vi "CRYTable Value Change.vi"(4 "Column":i32, 6 "Row":i32, 7 "TableVI":refnum<vi>, 8 "NewVal":string, 9 "OldVal":string, 10 "Index":i32, 11 "Type":enum16{"Curves", "Values", "Results", "WFM"}(ring)) -> ()   [LabVIEW 2013]
uses:
  Control/CRYTable Property.ctl
panel:
  in  "Table Property":T1 {"Precision" items=["Digits of precision", "Significant digits"]}
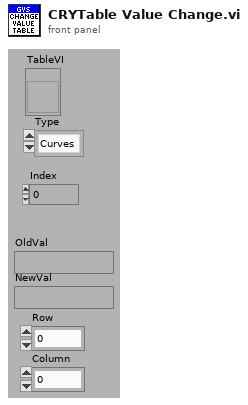
[diagram p1: front panel]
types:
  T1 = typedef "CRYTable Property.ctl" = cluster{"Reset All Columns":bool, "Transpose":bool, "Display Units":bool, "Notation":u16, "Digits":u16, "Precision":u16, "Hide Traling Zeros":bool, "Column Width":u16, "Row Header Width":u16, "Show vertical scroll bar":bool, "Show horizontal scroll bar":bool}
  T2 = enum16{"OK", "Yes", "YesNo", "YesNoCancel", "ReplaceAppend"}
  T3 = typedef "CRYData Cluster.ctl" = cluster{"Name":string, "Curve":cluster{"x":dbl, "y":dbl, "z":dbl}[], "X data":u16, "Y data":u16, "Z data":u16, "X axis":u16, "Y axis":u16, "Z axis":u16, "X unit":string, "Y unit":string, "Z unit":string, "X dB ref":dbl, "Y dB ref":dbl, "Z dB ref":dbl, "single val":bool, "protected":bool, "display X":bool, "display Y":bool, "display Z":bool, "Test Info":string, "Step No.":i32, "Plot Settings":cluster{"Color":u32, "Interpolation":u8, "Point Style":u8, "Line Style":u8, "Point Color":u32, "Line Width":u8, "Bar Plot Style":u8, "Fill To":i16}, "AutoProtect":bool}
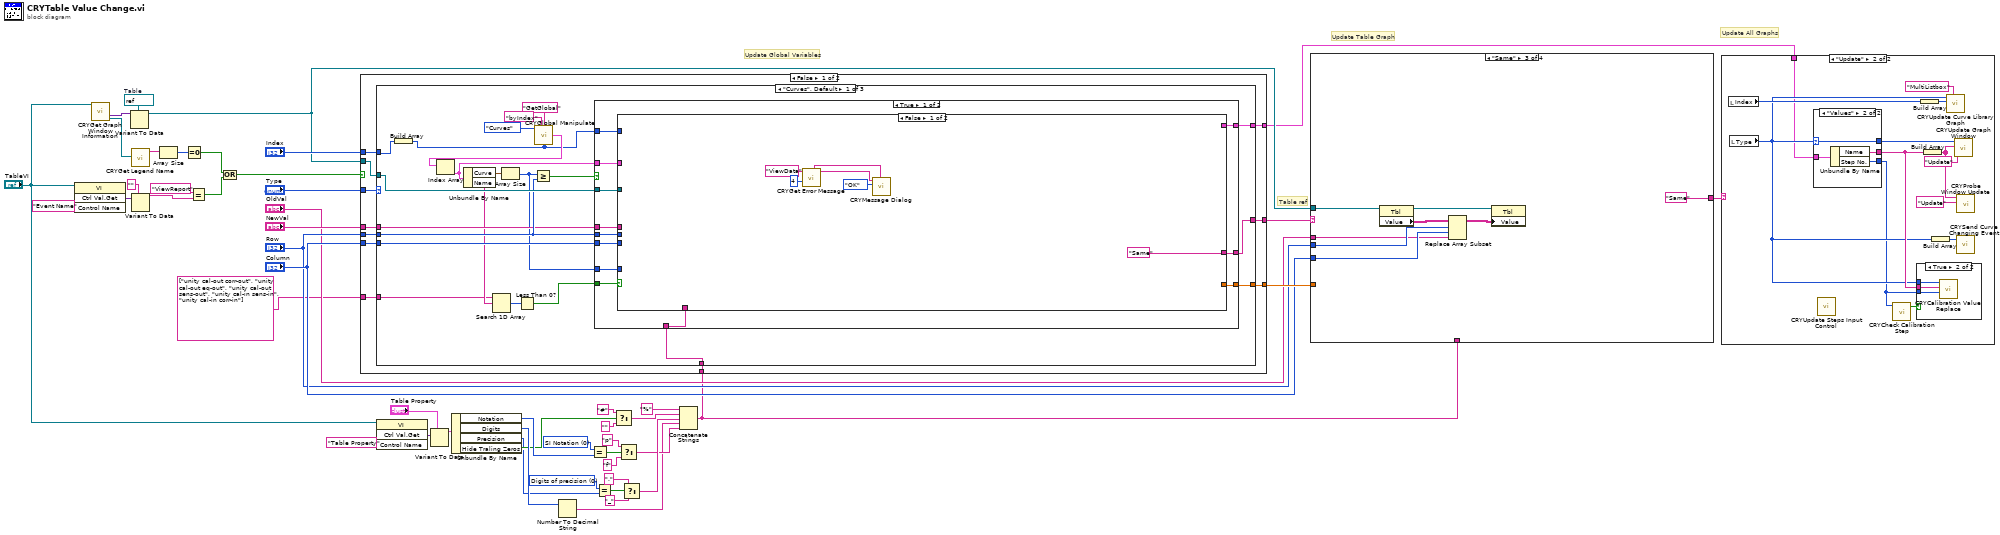
[diagram p0: block diagram]
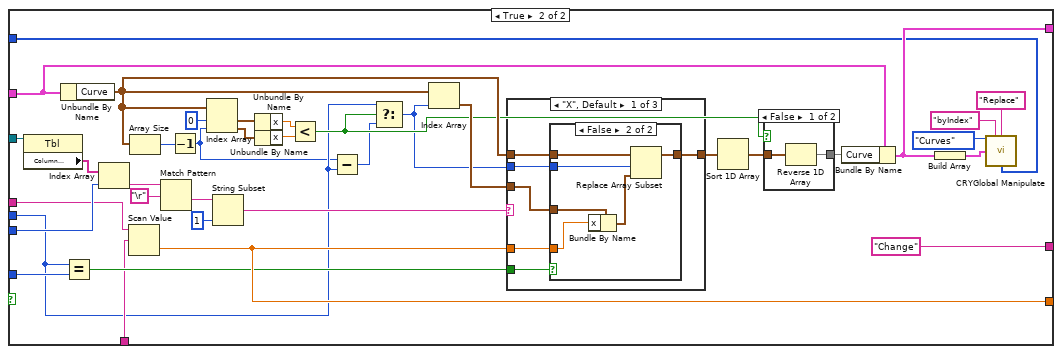
[diagram p2: hidden frame]
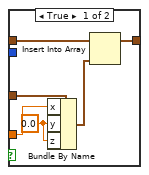
[diagram p4: hidden frame]
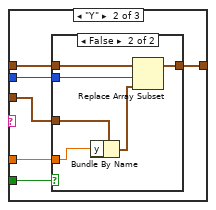
[diagram p5: hidden frame]
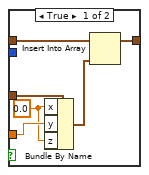
[diagram p6: hidden frame]
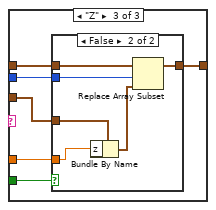
[diagram p7: hidden frame]
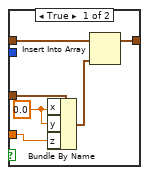
[diagram p8: hidden frame]
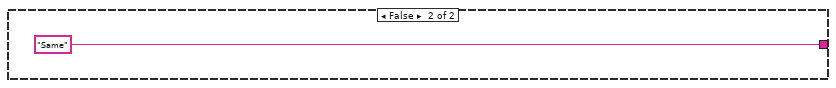
[diagram p9: hidden frame]
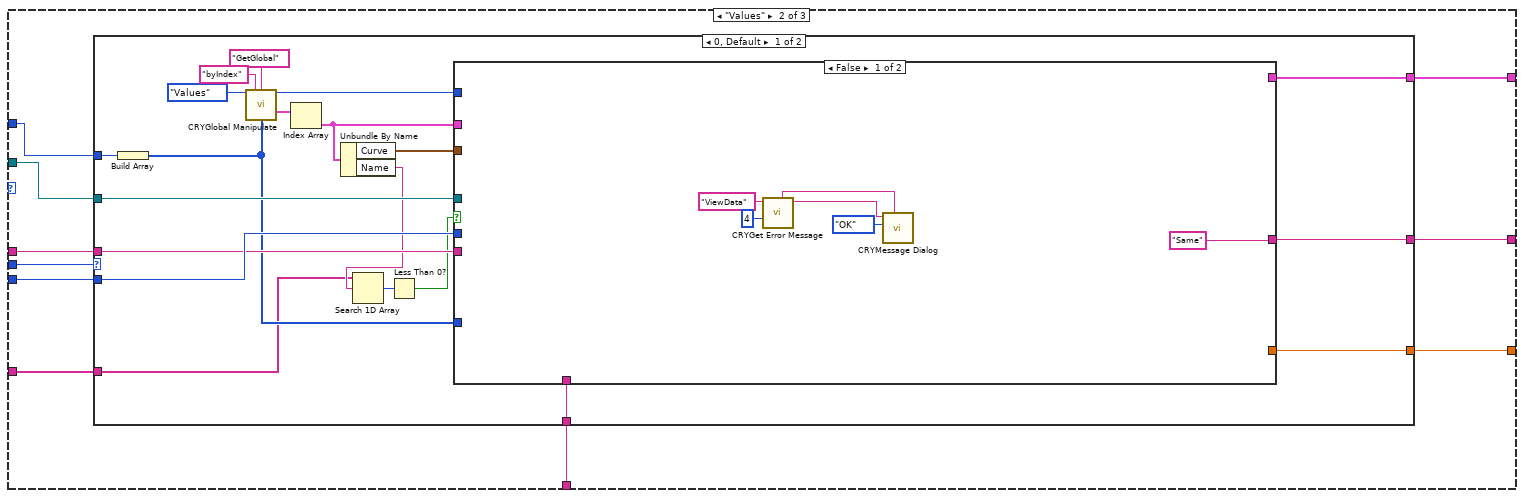
[diagram p10: hidden frame]
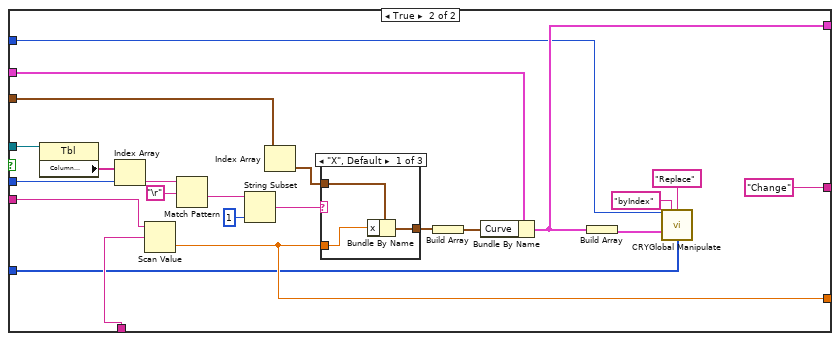
[diagram p11: hidden frame]
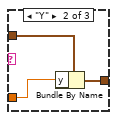
[diagram p12: hidden frame]
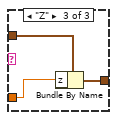
[diagram p13: hidden frame]
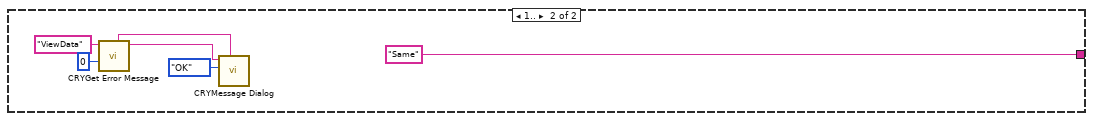
[diagram p14: hidden frame]
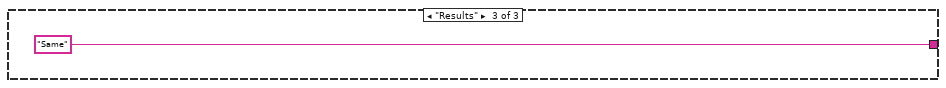
[diagram p15: hidden frame]
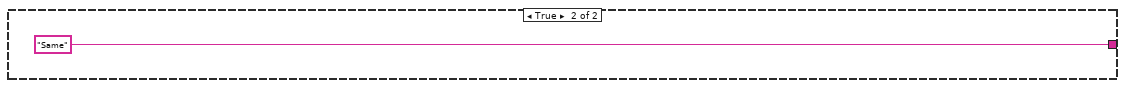
[diagram p16: hidden frame]
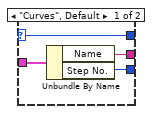
[diagram p19: hidden frame]
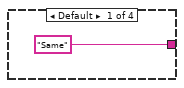
[diagram p20: hidden frame]
diagram:
  w31 = u16 0 items=["Digits of precision", "Significant digits"] ("Precision")
  w32 = u16 0 items=["SI Notation", "Floating point"] ("Notation")
  w48 = refnum<vi> refnum  # Table
  # "Table ref"
  # "Update All Graphs"
  # "Update Table Graph"
  # "Update Global Variables"
  n1 = invoke class="VI" method="Ctrl Val.Get"(reference="TableVI", "Control Name"="Event Name") -> ("Get Control Value Variant"=w14:variant)  [unwired: 2 in, 3 out]
  n2 = call "CRYGet Graph Window Information.vi"("pGraph VI In"="TableVI") -> ("Graph Control Ref Out"=w47:variant, "Legend Ref Out"=w11:refnum<vi>)  [unwired: 4 in, 9 out]
  n3 = Variant To Data(type=w48, Variant=w47) -> (data=w3:refnum<vi>)  [unwired: 1 in, 1 out]
  n4 = call "CRYGet Legend Name.vi"("MCListbox Refnum"=w11) -> ("Names Out"=w8:string[])  [unwired: 10 in]
  n5 = Variant To Data(type="" ("Control Name"), Variant=w14) -> (data=w10:string)  [unwired: 1 in, 1 out]
  n6 = Array Size(array=w8) -> (size(s)=w7:i32)
  n7 = Equal To 0?(x=w7) -> (x = 0?=w6:bool)
  n8 = Equal?(x="ViewReport", y=w10) -> (x = y?=w5:bool)
  n9 = Or(x=w6, y=w5) -> (x .or. y?=w4:bool)
  n10 = invoke class="VI" method="Ctrl Val.Get"(reference="TableVI", "Control Name"="Table Property") -> ("Get Control Value Variant"=w39:variant)  [unwired: 2 in, 3 out]
  n11 = Variant To Data(type="Table Property", Variant=w39) -> (data=w37:T1)  [unwired: 1 in, 1 out]
  n12 = Unbundle By Name(w37) -> ("Notation"=w35:u16, "Digits"=w36:u16, "Precision"=w33:u16, "Hide Traling Zeros"=w34:bool)
  n13 = Number To Decimal String(number=w36) -> (decimal integer string=w18:string)  [unwired: 1 in]
  n14 = Equal?(x=w32, y=w35) -> (x = y?=w29:bool)
  n15 = Equal?(x=w31, y=w33) -> (x = y?=w23:bool)
  n16 = Select(t="#" ("format string"), s=w34, f="" ("format string")) -> (s? t:f=w24:string)
  n17 = Select(t="p" ("string"), s=w29, f="f" ("string")) -> (s? t:f=w19:string)
  n18 = Select(t=".", s=w23, f="_") -> (s? t:f=w22:string)
  n19 = Concatenate Strings("%" ("string"), w24, w22, w18, w19) -> (w16:string)
  n20 = case shown="False" w4 {
    tunnel: [w61 _] -> w50
    tunnel: [w60 "Same" ("output string")] -> w49
    tunnel: w3 -> [w59 _]
    tunnel: "Column" -> [w58 _]
    tunnel: "Row" -> [w57 _]
    tunnel: "Type" -> [w56 _]
    tunnel: "Index" -> [w55 _]
    tunnel: "NewVal" -> [w54 _]
    tunnel: w16 -> [w53 _]
    tunnel: [w52 _] -> w2
    tunnel: string[] ["unity cal-out corr-out", "unity cal-out eq-out", "unity cal-out sens-out", "unity cal-in sens-in", "unity cal-in corr-in"] ("item tags") -> [w51 _]
    frame False {
      n21 = case shown="\"Curves\", Default" w56 {
        tunnel: w57 -> [w80 w204 _]
        tunnel: w58 -> [w83 w206 _]
        tunnel: w59 -> [w82 w205 _]
        tunnel: w55 -> [w74 w203 _]
        tunnel: [w79 w202 _] -> w61
        tunnel: [w78 w201 "Same" ("output string")] -> w60
        tunnel: w54 -> [w77 w200 _]
        tunnel: w53 -> [w75 w199 _]
        tunnel: [w71 w198 _] -> w52
        tunnel: w51 -> [w65 w197 _]
        frame "Curves", Default {
          n22 = Build Array(w74) -> (w67:i32[])
          n23 = call "CRYGlobal Manipulate.vi"("Type"=enum16{"Curves", "Values", "Results", "WFM"}."Curves", "sOption"="byIndex", "sAction"="GetGlobal", "nData"=w67) -> ("Curves Out"=w73:T3[])  [unwired: 5 in, 6 out]
          n24 = Index Array(array=w73) -> (element=w72:T3)  [unwired: 1 in]
          n25 = Unbundle By Name(w72) -> ("Curve"=w81:cluster{"x":dbl, "y":dbl, "z":dbl}[], "Name"=w66:string)
          n26 = Search 1D Array(1D array=w65, element=w66) -> (index of element=w64:i32)  [unwired: 1 in]
          n27 = Array Size(array=w81) -> (size(s)=w76:i32)
          n28 = Less Than 0?(x=w64) -> (x < 0?=w62:bool)
          n29 = Greater Or Equal?(x=w76, y=w80) -> (x >= y?=w63:bool)
          n30 = case shown="True" w63 {
            tunnel: w80 -> [w88 _]
            tunnel: w83 -> [w95 _]
            tunnel: w82 -> [w94 _]
            tunnel: [w93 _] -> w79
            tunnel: [w90 "Same" ("output string")] -> w78
            tunnel: w77 -> [w92 _]
            tunnel: w76 -> [w91 _]
            tunnel: w75 -> [w89 _]
            tunnel: w72 -> [w87 _]
            tunnel: w67 -> [w85 _]
            tunnel: [w86 _] -> w71
            tunnel: w62 -> [w84 _]
            frame True {
              n31 = case shown="False" w84 {
                tunnel: w95 -> [_ w137]
                tunnel: w94 -> [_ w133]
                tunnel: [_ w129] -> w93
                tunnel: w92 -> [_ w128]
                tunnel: w91 -> [_ w127]
                tunnel: ["Same" ("output string") "Change" ("output string")] -> w90
                tunnel: w89 -> [_ w124]
                tunnel: w88 -> [_ w113]
                tunnel: w87 -> [_ w105]
                tunnel: [_ w104] -> w86
                tunnel: w85 -> [_ w103]
                frame False {
                  n32 = call "CRYGet Error Message.vi"("Error No"=4, "Kind"="ViewData") -> ("Message"=w96:string, "Window Title"=w97:string)  [unwired: 4 in, 4 out]
                  n33 = call "CRYMessage Dialog.vi"("Window Title"=w97, "YesNoCancel"=T2."OK", "Message Content"=w96) -> ()  [unwired: 7 in, 2 out]
                }
                frame True {
                  n34 = property on="Property Node" class="Tbl"(reference=w133) -> ("Column Headers[]"=w138:string[])  [unwired: 1 in, 2 out]
                  n35 = Unbundle By Name(w105) -> ("Curve"=w123:cluster{"x":dbl, "y":dbl, "z":dbl}[])
                  n36 = Equal?(x=w113, y=w127) -> (x = y?=w126:bool)
                  n37 = Index Array(array=w138, index=w137) -> (element=w131:string)
                  n38 = Scan Value(string=w128, format string=w124) -> (value=w129:dbl)  [unwired: 1 in, 1 out]
                  n39 = Array Size(array=w123) -> (size(s)=w111:i32)
                  n40 = Match Pattern(string=w131, regular expression="\r") -> (after substring=w130:string)  [unwired: 1 in, 3 out]
                  n41 = Decrement(x=w111) -> (x-1=w109:i32)
                  n42 = Index Array(array=w123, index #1=0 ("index"), index #2=w109) -> (element #1=w121:cluster{"x":dbl, "y":dbl, "z":dbl}, element #2=w120:cluster{"x":dbl, "y":dbl, "z":dbl})
                  n43 = String Subset(string=w130, length (rest)=1 ("length (rest)")) -> (substring=w135:string)  [unwired: 1 in]
                  n44 = Unbundle By Name(w121) -> ("x"=w119:dbl)
                  n45 = Unbundle By Name(w120) -> ("x"=w118:dbl)
                  n46 = Less?(x=w119, y=w118) -> (x < y?=w114:bool)
                  n47 = Subtract(x=w109, y=w113) -> (x-y=w112:i32)
                  n48 = Select(t=w113, s=w114, f=w112) -> (s? t:f=w110:i32)
                  n49 = Index Array(array=w123, index=w110) -> (element=w134:cluster{"x":dbl, "y":dbl, "z":dbl})
                  n50 = case shown="\"X\", Default" w135 {
                    tunnel: w134 -> [w145 w163 w181]
                    tunnel: w129 -> [w147 w165 w183]
                    tunnel: w123 -> [w144 w162 w180]
                    tunnel: w110 -> [w143 w161 w179]
                    tunnel: [w142 w160 w178] -> w116
                    tunnel: w126 -> [w146 w164 w182]
                    frame "X", Default {
                      n51 = case shown="False" w146 {
                        tunnel: w147 -> [w153 w159]
                        tunnel: w145 -> [w152 w158]
                        tunnel: w144 -> [w150 w157]
                        tunnel: [w148 w155] -> w142
                        tunnel: w143 -> [_ w154]
                        frame True {
                          w151 = 0.0 ("y")
                          n52 = Bundle By Name(cluster=w152, "x"=w153, "y"=w151, "z"=w151) -> (w149:cluster{"x":dbl, "y":dbl, "z":dbl})
                          n53 = Insert Into Array(array=w150, new element=w149) -> (w148:cluster{"x":dbl, "y":dbl, "z":dbl}[])  [unwired: 1 in]
                        }
                        frame False {
                          n54 = Bundle By Name(cluster=w158, "x"=w159) -> (w156:cluster{"x":dbl, "y":dbl, "z":dbl})
                          n55 = Replace Array Subset(array=w157, new element=w156, index=w154) -> (w155:cluster{"x":dbl, "y":dbl, "z":dbl}[])
                        }
                      }
                    }
                    frame "Y" {
                      n56 = case shown="False" w164 {
                        tunnel: w165 -> [w167 w172]
                        tunnel: w163 -> [w171 w177]
                        tunnel: w162 -> [w170 w176]
                        tunnel: [w168 w174] -> w160
                        tunnel: w161 -> [_ w173]
                        frame True {
                          w166 = 0.0 ("x")
                          n57 = Bundle By Name(cluster=w171, "x"=w166, "y"=w167, "z"=w166) -> (w169:cluster{"x":dbl, "y":dbl, "z":dbl})
                          n58 = Insert Into Array(array=w170, new element=w169) -> (w168:cluster{"x":dbl, "y":dbl, "z":dbl}[])  [unwired: 1 in]
                        }
                        frame False {
                          n59 = Bundle By Name(cluster=w177, "y"=w172) -> (w175:cluster{"x":dbl, "y":dbl, "z":dbl})
                          n60 = Replace Array Subset(array=w176, new element=w175, index=w173) -> (w174:cluster{"x":dbl, "y":dbl, "z":dbl}[])
                        }
                      }
                    }
                    frame "Z" {
                      n61 = case shown="False" w182 {
                        tunnel: w183 -> [w184 w195]
                        tunnel: w181 -> [w189 w194]
                        tunnel: w180 -> [w188 w193]
                        tunnel: [w186 w191] -> w178
                        tunnel: w179 -> [_ w190]
                        frame True {
                          w185 = 0.0 ("y")
                          n62 = Bundle By Name(cluster=w189, "x"=w185, "y"=w185, "z"=w184) -> (w187:cluster{"x":dbl, "y":dbl, "z":dbl})
                          n63 = Insert Into Array(array=w188, new element=w187) -> (w186:cluster{"x":dbl, "y":dbl, "z":dbl}[])  [unwired: 1 in]
                        }
                        frame False {
                          n64 = Bundle By Name(cluster=w194, "z"=w195) -> (w192:cluster{"x":dbl, "y":dbl, "z":dbl})
                          n65 = Replace Array Subset(array=w193, new element=w192, index=w190) -> (w191:cluster{"x":dbl, "y":dbl, "z":dbl}[])
                        }
                      }
                    }
                  }
                  n66 = Sort 1D Array(array=w116) -> (sorted array=w115:cluster{"x":dbl, "y":dbl, "z":dbl}[])
                  n67 = case shown="False" w114 {
                    tunnel: w115 -> [w140 w141]
                    tunnel: [w139 w141] -> w117
                    frame False {
                      n68 = Reverse 1D Array(array=w140) -> (reversed array=w139:cluster{"x":dbl, "y":dbl, "z":dbl}[])
                    }
                    frame True {
                    }
                  }
                  n69 = Bundle By Name(cluster=w105, "Curve"=w117) -> (w104:T3)
                  n70 = Build Array(w104) -> (w106:T3[])
                  n71 = call "CRYGlobal Manipulate.vi"("Type"=enum16{"Curves", "Values", "Results", "WFM"}."Curves", "sOption"="byIndex", "sAction"="Replace", "Curves"=w106, "nData"=w103) -> ()  [unwired: 4 in, 7 out]
                }
              }
            }
            frame False {
            }
          }
        }
        frame "Values" {
          n72 = case shown="0, Default" w204 {
            tunnel: w206 -> [w226 _]
            tunnel: w205 -> [w224 _]
            tunnel: w203 -> [w219 _]
            tunnel: [w223 _] -> w202
            tunnel: [w222 "Same" ("output string")] -> w201
            tunnel: w200 -> [w221 _]
            tunnel: w199 -> [w220 _]
            tunnel: [w216 _] -> w198
            tunnel: w197 -> [w208 _]
            frame 0, Default {
              n73 = Build Array(w219) -> (w211:i32[])
              n74 = call "CRYGlobal Manipulate.vi"("Type"=enum16{"Curves", "Values", "Results", "WFM"}."Values", "sOption"="byIndex", "sAction"="GetGlobal", "nData"=w211) -> ("Type out"=w213:enum16{"Curves", "Values", "Results", "WFM"}, "Values Out"=w218:T3[])  [unwired: 5 in, 5 out]
              n75 = Index Array(array=w218) -> (element=w217:T3)  [unwired: 1 in]
              n76 = Unbundle By Name(w217) -> ("Curve"=w225:cluster{"x":dbl, "y":dbl, "z":dbl}[], "Name"=w209:string)
              n77 = Search 1D Array(1D array=w208, element=w209) -> (index of element=w210:i32)  [unwired: 1 in]
              n78 = Less Than 0?(x=w210) -> (x < 0?=w207:bool)
              n79 = case shown="False" w207 {
                tunnel: w226 -> [_ w254]
                tunnel: w225 -> [_ w251]
                tunnel: w224 -> [_ w249]
                tunnel: [_ w243] -> w223
                tunnel: ["Same" ("output string") "Change" ("output string")] -> w222
                tunnel: w221 -> [_ w241]
                tunnel: w220 -> [_ w240]
                tunnel: w217 -> [_ w237]
                tunnel: [_ w236] -> w216
                tunnel: w213 -> [_ w235]
                tunnel: w211 -> [_ w234]
                frame False {
                  n80 = call "CRYGet Error Message.vi"("Error No"=4, "Kind"="ViewData") -> ("Message"=w227:string, "Window Title"=w228:string)  [unwired: 4 in, 4 out]
                  n81 = call "CRYMessage Dialog.vi"("Window Title"=w228, "YesNoCancel"=T2."OK", "Message Content"=w227) -> ()  [unwired: 7 in, 2 out]
                }
                frame True {
                  n82 = property on="Property Node" class="Tbl"(reference=w249) -> ("Column Headers[]"=w255:string[])  [unwired: 1 in, 2 out]
                  n83 = Index Array(array=w255, index=w254) -> (element=w247:string)
                  n84 = Scan Value(string=w241, format string=w240) -> (value=w243:dbl)  [unwired: 1 in, 1 out]
                  n85 = Match Pattern(string=w247, regular expression="\r") -> (after substring=w246:string)  [unwired: 1 in, 3 out]
                  n86 = String Subset(string=w246, length (rest)=1 ("length (rest)")) -> (substring=w252:string)  [unwired: 1 in]
                  n87 = Index Array(array=w251) -> (element=w250:cluster{"x":dbl, "y":dbl, "z":dbl})  [unwired: 1 in]
                  n88 = case shown="\"X\", Default" w252 {
                    tunnel: w250 -> [w258 w261 w264]
                    tunnel: w243 -> [w257 w260 w263]
                    tunnel: [w256 w259 w262] -> w245
                    frame "X", Default {
                      n89 = Bundle By Name(cluster=w258, "x"=w257) -> (w256:cluster{"x":dbl, "y":dbl, "z":dbl})
                    }
                    frame "Y" {
                      n90 = Bundle By Name(cluster=w261, "y"=w260) -> (w259:cluster{"x":dbl, "y":dbl, "z":dbl})
                    }
                    frame "Z" {
                      n91 = Bundle By Name(cluster=w264, "z"=w263) -> (w262:cluster{"x":dbl, "y":dbl, "z":dbl})
                    }
                  }
                  n92 = Build Array(w245) -> (w244:cluster{"x":dbl, "y":dbl, "z":dbl}[])
                  n93 = Bundle By Name(cluster=w237, "Curve"=w244) -> (w236:T3)
                  n94 = Build Array(w236) -> (w238:T3[])
                  n95 = call "CRYGlobal Manipulate.vi"("Type"=w235, "sOption"="byIndex", "sAction"="Replace", "Values"=w238, "nData"=w234) -> ()  [unwired: 4 in, 7 out]
                }
              }
            }
            frame 1.. {
              n96 = call "CRYGet Error Message.vi"("Error No"=0, "Kind"="ViewData") -> ("Message"=w265:string, "Window Title"=w266:string)  [unwired: 4 in, 4 out]
              n97 = call "CRYMessage Dialog.vi"("Window Title"=w266, "YesNoCancel"=T2."OK", "Message Content"=w265) -> ()  [unwired: 7 in, 2 out]
            }
          }
        }
        frame "Results" {
        }
      }
    }
    frame True {
    }
  }
  n98 = case shown="\"Same\"" w49 {
    tunnel: w3 -> [_ w280 w289 _]
    tunnel: "Row" -> [_ w279 w288 _]
    tunnel: "Column" -> [_ w278 w287 _]
    tunnel: w50 -> [_ w277 _ _]
    tunnel: "OldVal" -> [_ _ w286 _]
    tunnel: ["Same" ("sAction") "Update" ("sAction") "Same" ("sAction") "Update" ("sAction")] -> w40
    tunnel: w16 -> [_ w274 _ _]
    frame Default {
    }
    frame "Change" {
      n99 = Format Value(format string=w274, value (0)=w277) -> (output string=w276:string)  [unwired: 1 in]
      n100 = property on="Property Node" class="Tbl"(reference=w280) -> (reference out=w281:refnum<vi>, "Value"=w283:string[][])  [unwired: 1 in, 1 out]
      n101 = Replace Array Subset(array=w283, new element=w276, index (row)=w279, index (col)=w278) -> (w282:string[][])
      n102 = property on="Property Node" class="Tbl"(reference=w281, "Value"=w282) -> ()  [unwired: 1 in, 2 out]
    }
    frame "Same" {
      n103 = property on="Property Node" class="Tbl"(reference=w289) -> (reference out=w284:refnum<vi>, "Value"=w291:string[][])  [unwired: 1 in, 1 out]
      n104 = Replace Array Subset(array=w291, new element=w286, index (row)=w288, index (col)=w287) -> (w290:string[][])
      n105 = property on="Property Node" class="Tbl"(reference=w284, "Value"=w290) -> ()  [unwired: 1 in, 2 out]
    }
    frame "Replot" {
    }
  }
  n106 = case shown="\"Update\"" w40 {
    tunnel: w2 -> [_ w293]
    frame "Same", Default {
    }
    frame "Update" {
      n107 = local read "Index"() -> (w300:i32)
      n108 = local read "Type"() -> (w298:enum16{"Curves", "Values", "Results", "WFM"})
      n109 = case shown="\"Values\"" w298 {
        selector: w298 -> [w311 w315]
        tunnel: [w312 w316] -> w302
        tunnel: [w311 w315] -> w301
        tunnel: [w310 w314] -> w294
        tunnel: w293 -> [w309 w313]
        frame "Curves", Default {
          n110 = Unbundle By Name(w309) -> ("Name"=w312:string, "Step No."=w310:i32)
        }
        frame "Values" {
          n111 = Unbundle By Name(w313) -> ("Name"=w316:string, "Step No."=w314:i32)
        }
      }
      n112 = call "CRYUpdate Steps Input Control.vi"() -> ()  [unwired: 12 in]
      n113 = call "CRYCheck Calibration Step.vi"("Step No"=w294) -> ("Is Calibration?"=w295:bool)  [unwired: 9 in, 1 out]
      n114 = case shown="True" w295 {
        tunnel: w298 -> [_ w308]
        tunnel: w302 -> [_ w307]
        tunnel: w294 -> [_ w306]
        frame False {
        }
        frame True {
          n115 = call "CRYCalibration Value Replace.vi"("Step No."=w306, "Corr/EQ/Sens Name"=w307, "Type"=w308) -> ()  [unwired: 9 in]
        }
      }
      n116 = Build Array(w300) -> (w297:i32[])
      n117 = Build Array(w302) -> (w304:string[])
      n118 = Build Array(w298) -> (w303:enum16{"Curves", "Values", "Results", "WFM"}[])
      n119 = call "CRYUpdate Curve Library Graph.vi"("sOption 1"="MultiListbox" ("sOption"), "Index"=w297, "Type"=w298) -> ()  [unwired: 9 in]
      n120 = call "CRYUpdate Graph Window.vi"("sOption"="Update", "Del/Update Names"=w304, "Type"=w301) -> ()  [unwired: 1 in, 8 out]
      n121 = call "CRYSend Curve Changing Event.vi"("Type"=w303) -> ()  [unwired: 11 out]
      n122 = call "CRYProbe Window Update.vi"("sAction"="Update", "Names"=w304) -> ()  [unwired: 2 in, 8 out]
    }
  }
